vi "NicmosMaskListToSquareMaskList.vi"(3 "Mask In [8x128x128]":bool[][][](array[boolean]), 9 "error in (no error)":errorcluster caption="entrée d'erreur") -> (0 "Mask Out [8x128x128]":bool[][][](array[boolean]), 6 "error out":errorcluster caption="sortie d'erreur")   [LabVIEW 2009]
uses:
  NicmosGlobal.vi
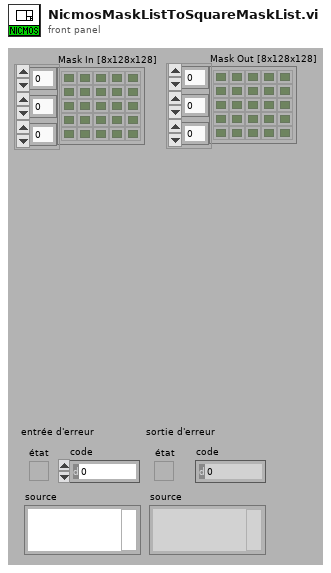
[diagram p1: front panel]
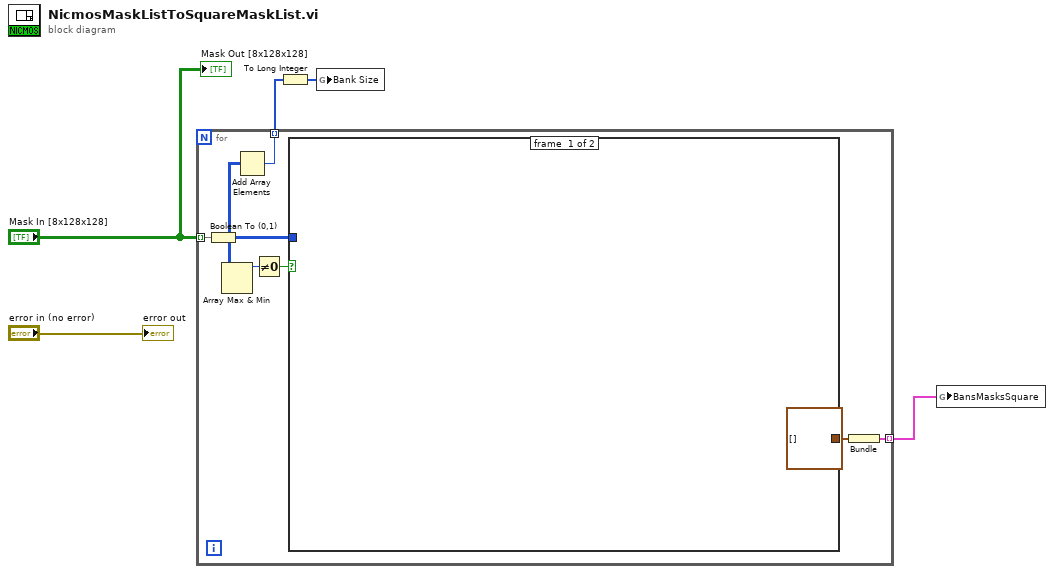
[diagram p0: block diagram]
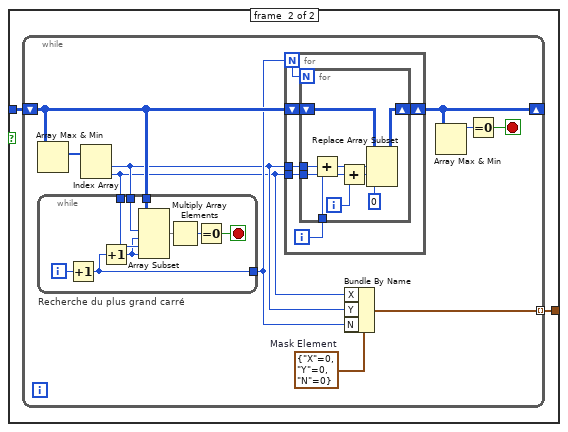
[diagram p2: hidden frame]
diagram:
  n1 = for {
    tunnel: "Mask In [8x128x128]" -> [w12] mode=indexing
    tunnel: [w7] -> w1 mode=indexing
    tunnel: [w6] -> w4 mode=indexing
    n2 = Boolean To (0,1)(Boolean=w12) -> (0, 1=w10:i16[][])
    n3 = Array Max & Min(array=w10) -> (max value=w11:i16)  [unwired: 3 out]
    n4 = Add Array Elements(numeric array=w10) -> (sum=w6:i16)
    n5 = Not Equal To 0?(x=w11) -> (x != 0?=w9:bool)
    n6 = case shown="True" w9 {
      tunnel: w10 -> [_ w15]
      tunnel: [cluster{"X":i32, "Y":i32, "N":i32}[] [] w14] -> w8
      frame #0 {
      }
      frame #1 {
        n7 = while {
          shift-right: [w17] -> _
          shift-left: w15 -> [w23]
          tunnel: [w18] -> w14 mode=indexing
          stop <- w24 stop-if-true
          w22 = cluster{"X":i32, "Y":i32, "N":i32} {"X"=0, "Y"=0, "N"=0}  # Mask Element
          n8 = Array Max & Min(array=w23) -> (max index (indices)=w25:i32[])  [unwired: 3 out]
          n9 = Index Array(array=w25) -> (element #1=w20:i32, element #2=w19:i32)  [unwired: 2 in]
          n10 = while "Recherche du plus grand carré" {
            tunnel: w23 -> [w48]
            tunnel: w20 -> [w47]
            tunnel: w19 -> [w46]
            tunnel: [w45] -> w21
            i -> [w49]
            stop <- w42 stop-if-true
            n11 = Increment(x=w49) -> (x+1=w45:i32)
            n12 = Increment(x=w45) -> (x+1=w41:i32)
            n13 = Array Subset(array=w48, index (row)=w47, length (row)=w41, index (col)=w46, length (col)=w41) -> (w44:i16[][])
            n14 = Multiply Array Elements(1:w44) -> (0:w43:i16)
            n15 = Equal To 0?(x=w43) -> (x = 0?=w42:bool)
          }
          n16 = for {
            N: w21 -> [w29]
            tunnel: w20 -> [w31]
            tunnel: w19 -> [w30]
            shift-right: [w27] -> w17
            shift-left: w23 -> [w28]
            i -> [w26]
            n17 = for {
              N: w29 -> [_]
              tunnel: w31 -> [w38]
              tunnel: w30 -> [w35]
              shift-right: [w39] -> w27
              shift-left: w28 -> [w40]
              tunnel: w26 -> [w33]
              i -> [w34]
              n18 = Add(x=w38, y=w33) -> (x+y=w37:i32)
              n19 = Add(x=w35, y=w34) -> (x+y=w36:i32)
              n20 = Replace Array Subset(array=w40, new element=i16 0 ("nouvel élt/sous-tableau"), index (row)=w37, index (col)=w36) -> (w39:i16[][])
            }
          }
          n21 = Bundle By Name(cluster=w22, "X"=w19, "Y"=w20, "N"=w21) -> (w18:cluster{"X":i32, "Y":i32, "N":i32})
          n22 = Array Max & Min(array=w17) -> (max value=w16:i16)  [unwired: 3 out]
          n23 = Equal To 0?(x=w16) -> (x = 0?=w24:bool)
        }
      }
    }
    n24 = Bundle(w8) -> (w7:cluster{cluster{"X":i32, "Y":i32, "N":i32}[]})  [unwired: 1 in]
  }
  n25 = To Long Integer(number=w4) -> (32bit integer=w3:i32[])
  n26 = global write "NicmosGlobal.vi" "Bank Size"(w3) -> ()
  n27 = global write "NicmosGlobal.vi" "BansMasksSquare"(w1) -> ()
  "error out" <- "error in (no error)"
  "Mask Out [8x128x128]" <- "Mask In [8x128x128]"
